vi "Set Edit Field.vi"(8 "error in (no error)":errorcluster, 10 "Edit Field (0: OFF)":u32(ring) items=["OFF", "PRI", "SEC", "FREQ"], 11 "VISA resource name":refnum<visa-resource-name>) -> (0 "error out":errorcluster, 3 "VISA resource name out":refnum<visa-resource-name>)   [LabVIEW 2011, in "Fluke 5XXX Series Multicalibrators.lvlib"]
doc: "This VI sets the edit field to the primary, secondary or frequency field.\n\nNote:\n\nThis VI is available only for instrument models 5500A and 5520A."
uses:
  Fluke 5XXX Series Multicalibrators.lvlib
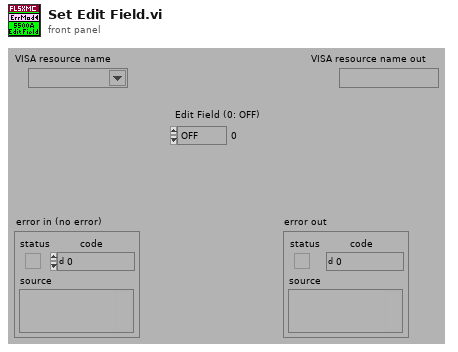
[diagram p1: front panel]
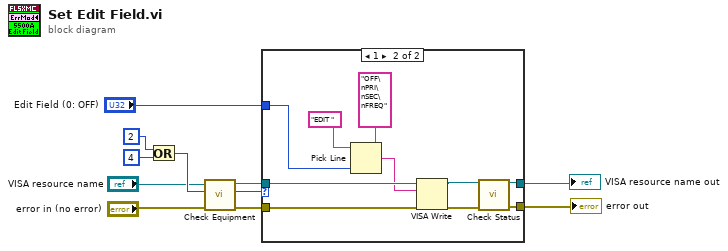
[diagram p0: block diagram]
diagram:
  n1 = Or(x=2 ("Numeric"), y=4 ("Numeric")) -> (x .or. y?=w8:i32)
  n2 = call "Check Equipment.vi"("error in (no error)"="error in (no error)", "Bit Mask"=w8, "VISA resource name"="VISA resource name") -> ("error out"=w11:errorcluster, "Present?"=w10:u32, "VISA resource name out"=w9:refnum<visa-resource-name>)  [unwired: 6 in]
  n3 = case shown="1" w10 {
    tunnel: "Edit Field (0: OFF)" -> [_ w18]
    tunnel: [w12 w14] -> w1
    tunnel: w11 -> [w13 w21]
    tunnel: w9 -> [w12 w20]
    tunnel: [w13 w17] -> w2
    frame 0, Default {
    }
    frame 1 {
      n4 = Pick Line(string ("")="EDIT " ("Reset Command"), multi-line string="OFF\nPRI\nSEC\nFREQ", line index=w18) -> (output string=w19:string)
      n5 = VISA Write(VISA resource name=w20, write buffer=w19, error in (no error)=w21) -> (VISA resource name out=w15:refnum<visa-resource-name>, error out=w16:errorcluster)  [unwired: 1 out]
      n6 = call "Check Status.vi"("VISA resource name"=w15, "error in (no error)"=w16) -> ("VISA resource name out"=w14:refnum<visa-resource-name>, "error out"=w17:errorcluster)  [unwired: 12 in]
    }
  }
  "VISA resource name out" <- w1
  "error out" <- w2
